vi "4_2.vi"() -> ()   [LabVIEW 2020]
panel:
  out "Output":string[](array[string])
  in  "Delimeters":string
  out "Output":string[](array[string])
  in  "Input":string
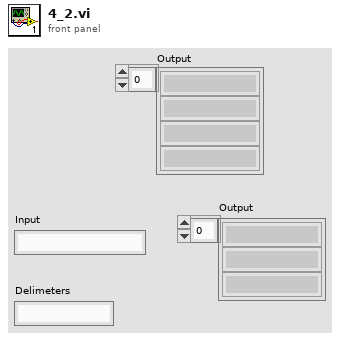
[diagram p1: front panel]
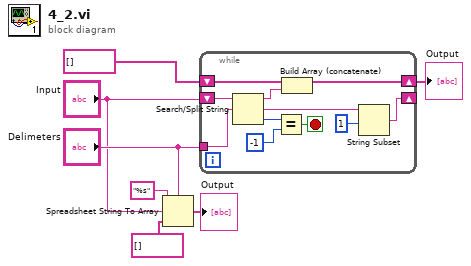
[diagram p0: block diagram]
diagram:
  n1 = Spreadsheet String To Array(delimiter (Tab)="Delimeters", format string="%s", spreadsheet string="Input", array type (2D Dbl)=string[] []) -> (array=→"Output":string[])
  n2 = while {
    tunnel: "Delimeters" -> [w17]
    shift-right: [w10] -> _
    shift-left: "Input" -> [w18]
    shift-right: [w15] -> w7
    shift-left: string[] [] -> [w14]
    stop <- w12 stop-if-true
    n3 = Search/Split String(string=w18, search string/char (-)=w17) -> (substring before match=w16:string, match + rest of string=w11:string, offset of match=w13:i32)  [unwired: 1 in]
    n4 = Equal?(x=w13, y=-1) -> (x = y?=w12:bool)
    n5 = Build Array (concatenate)(w14, w16) -> (w15:string[])
    n6 = String Subset(string=w11, offset (0)=1) -> (substring=w10:string)  [unwired: 1 in]
  }
  "Output" <- w7
